vi "Asylum_Driver_XYMetersToVoltagePolymorphic.vi"   [LabVIEW 2019]
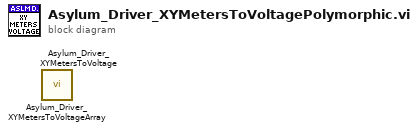
[diagram p0: block diagram]
diagram:
  n1 = call "Asylum_Driver_XYMetersToVoltageArray.vi"() -> ()  [unwired: 8 in, 4 out]
  n2 = call "Asylum_Driver_XYMetersToVoltage.vi"() -> ()  [unwired: 8 in, 4 out]
